vi "Out_S7F6.vi"(8 "error in (no error)":errorcluster, 10 "S7F6":T1, 11 "S7 Message Class in":refnum<class "S7 Message Class.lvclass">) -> (0 "error out":errorcluster, 3 "S7 Message Class out":refnum<class "S7 Message Class.lvclass">)   [LabVIEW 2020, in "SECS Communication.lvlib" / "S7 Message Class.lvclass"]
uses:
  S7 Message Class.lvclass
  D:/Dropbox/SECS/LabVIEW Code/Com/SECS Communication/SECS-II Class/SECS-II Class.lvclass
  S7F6.ctl
  SECS-II Class/Data Message_List.vi
  SECS-II Class/Data Message_ASCII.vi
  SECS-II Class/Data Message_Binary.vi
  S7 Message Class.lvclass/S7 Message Class.ctl
  SECS-II Class/SECS-II Class.lvclass
  D:/Dropbox/SECS/LabVIEW Code/Com/SECS Communication/S7 Message Class/S7 Message Class.lvclass
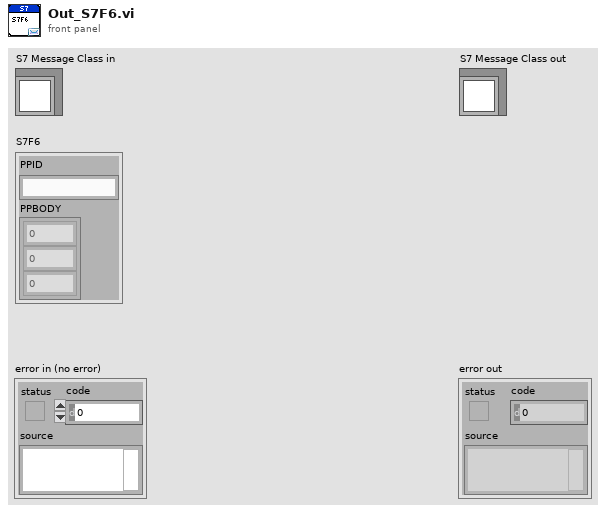
[diagram p1: front panel]
types:
  T1 = typedef "SECS Communication.lvlib/S7 Message Class.lvclass/S7F6.ctl" = cluster{"PPID":string, "PPBODY":u8[]}
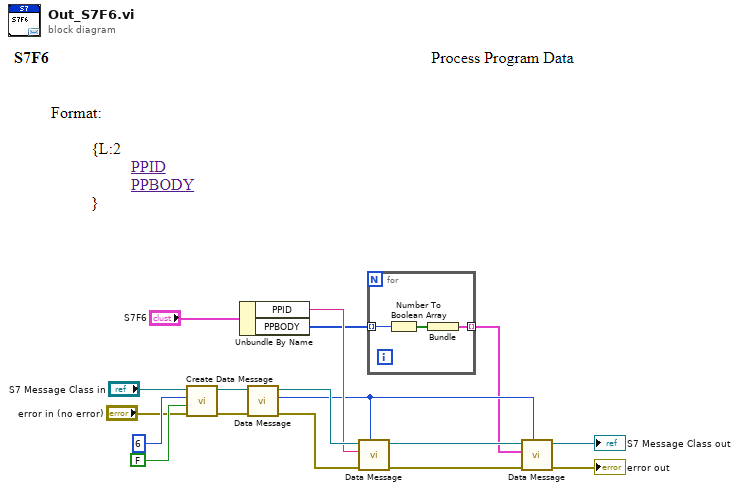
[diagram p0: block diagram]
diagram:
  n1 = call "Create Data Message.vi"("error in (no error)"="error in (no error)", "W-Bit"=FALSE, "Function"=u8 6, "SECS-II Class in"="S7 Message Class in") -> ("error out"=w14:errorcluster, "SECS-II Class out"=w15:refnum<class "S7 Message Class.lvclass">)  [unwired: 6 in]
  n2 = Unbundle By Name("S7F6") -> ("PPID"=w8:string, "PPBODY"=w2:u8[])
  n3 = call-poly "Data Message.vi"("error in"=w14, "SECS-II Class in"=w15) -> ("error out"=w10:errorcluster, "Index"=w3:i32, "SECS-II Class out"=w11:refnum<class "S7 Message Class.lvclass">)  [unwired: 7 in]
  n4 = call-poly "Data Message.vi"("Parent Index"=w3, "error in"=w10, "Data"=w8, "SECS-II Class in"=w11) -> ("error out"=w6:errorcluster, "SECS-II Class out"=w7:refnum<class "S7 Message Class.lvclass">)  [unwired: 6 in]
  n5 = for {
    tunnel: w2 -> [w20] mode=indexing
    tunnel: [w18] -> w1 mode=indexing
    n6 = Number To Boolean Array(number=w20) -> (Boolean array=w19:bool[])
    n7 = Bundle("Boolean array"=w19) -> (w18:cluster{"Boolean array":bool[]})  [unwired: 1 in]
  }
  n8 = call-poly "Data Message.vi"("Parent Index"=w3, "error in"=w6, "Data Cluster"=w1, "SECS-II Class in"=w7) -> ("error out"=→"error out":errorcluster, "SECS-II Class out"=→"S7 Message Class out":refnum<class "S7 Message Class.lvclass">)  [unwired: 6 in]
